vi "Wave2D_Init Data_BC_Extrapolation.vi"(10 "start?":bool=TRUE, 11 "Value":dbl[][](array[numeric])) -> (3 "Extrapolated Value":dbl[](array[numeric]))   [LabVIEW 2017, in "NI_PDE.lvlib"]
uses:
  <vilib>/gmath/NI_PDE.lvlib
  <vilib>/Analysis/1siggen.llb/Ramp Pattern by Samples.vi
  <vilib>/gmath/NI_Gmath.lvlib
  <vilib>/Analysis/NI_AALBase.lvlib
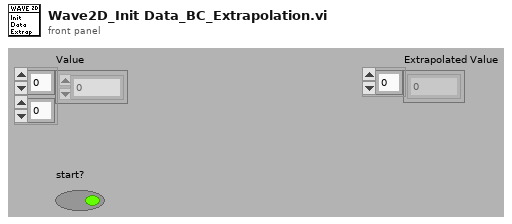
[diagram p1: front panel]
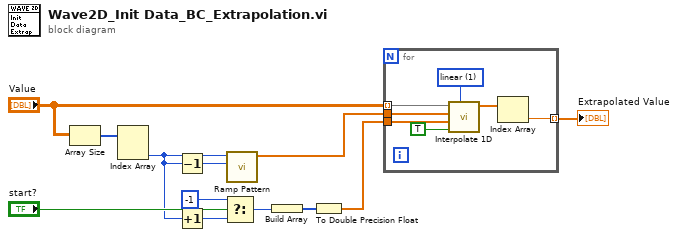
[diagram p0: block diagram]
diagram:
  n1 = Array Size(array="Value") -> (size(s)=w12:i32[])
  n2 = Index Array(array=w12) -> (element #2=w1:i32)  [unwired: 2 in, 1 out]
  n3 = Decrement(x=w1) -> (x-1=w2:i32)
  n4 = Increment(x=w1) -> (x+1=w7:i32)
  n5 = Select(t=-1, s="start?", f=w7) -> (s? t:f=w5:i32)
  n6 = call-poly <vilib>:"Ramp Pattern.vi"("end"=w2, "samples"=w1) -> ("Ramp Pattern"=w9:dbl[])  [unwired: 8 in, 1 out]
  n7 = Build Array(w5) -> (w4:i32[])
  n8 = To Double Precision Float(number=w4) -> (double precision float=w3:dbl[])
  n9 = for {
    tunnel: "Value" -> [w19] mode=indexing
    tunnel: [w17] -> w10 mode=indexing
    tunnel: w9 -> [w16]
    tunnel: w3 -> [w15]
    w13 = 1 items=["nearest", "linear", "spline", "cubic Hermite", "Lagrange"] ("method")
    n10 = call <vilib>:"Interpolate 1D.vi"("method"=w13, "X is monotonic"=TRUE, "xi"=w15, "X"=w16, "Y"=w19) -> ("yi"=w18:dbl[])  [unwired: 1 in, 5 out]
    n11 = Index Array(array=w18) -> (element=w17:dbl)  [unwired: 1 in]
  }
  "Extrapolated Value" <- w10
